vi "Icons.vi"() -> (4 "Selected":i32=38, 6 "Non Selected":i32=37)   [LabVIEW 2021, in "Packager Helpers.lvlib"]
uses:
  Packager Helpers.lvlib
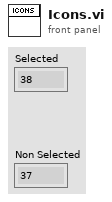
[diagram p1: front panel]
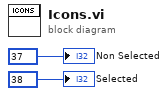
[diagram p0: block diagram]
diagram:
  "Non Selected" <- 37
  "Selected" <- 38
